vi "myRIO v1.0 Reset Encoder.vi"(8 "error in (no error)":errorcluster, 10 "Channel":T1, 11 "myRIO Ref In":T2) -> (0 "error out":errorcluster, 3 "myRIO Ref Out":T2)   [LabVIEW 2021]
uses:
  <vilib>/myRIO/Common/Instrument Driver Framework/Utilities/typedefs/myRIO v1.0 Reference.ctl
  <vilib>/myRIO/Common/Instrument Driver Framework/Utilities/typedefs/Generic FPGA Reference.ctl
  <vilib>/myRIO/Common/Instrument Driver Framework/myRIO v1.0/Encoder/typedefs/Encoder Channels Enum.ctl
  <vilib>/myRIO/Common/Instrument Driver Framework/myRIO v1.0/Encoder/typedefs/Encoder Channels FPGA Reference.ctl
  <vilib>/rvi/errors/niLvFpgaAdjustHostInterfaceError.vi
  <vilib>/rvi/interface/nirviReadWriteControl/nirviReadWriteControl.xnode
  <vilib>/rvi/interface/Simulation/niFpgaSimulationCallBeginRW.vi
  NiFpgaLv.dll
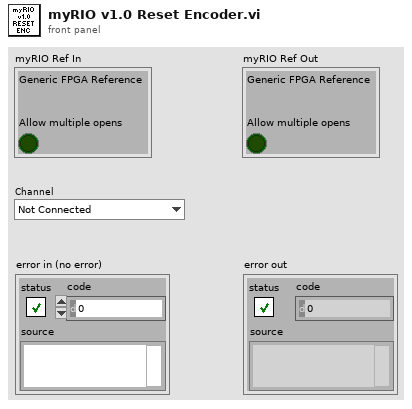
[diagram p1: front panel]
types:
  T1 = typedef "Encoder Channels Enum.ctl" = enum16{"Not Connected", "C/ENC0", "C/ENC1", "A/ENC", "A/ENC0", "A/ENC1", "A/ENC2", "A/ENC3", "A/ENC4", "A/ENC5", "A/ENC6", "A/ENC7", "A/ENC8", "A/ENC9", "B/ENC", "B/ENC0", "B/ENC1", "B/ENC2", "B/ENC3", "B/ENC4", "B/ENC5", "B/ENC6", "B/ENC7", "B/ENC8", "B/ENC9", "DIO/ENC0", "DIO/ENC1", "DIO/ENC2", "DIO/ENC3", "DIO/ENC4"}
  T2 = typedef "myRIO v1.0 Reference.ctl" = cluster{"Generic FPGA Reference":T3, "Allow multiple opens":bool}
  T3 = typedef "Generic FPGA Reference.ctl" = refnum<k20>
  T4 = typedef "Encoder Channels FPGA Reference.ctl" = refnum<k20>
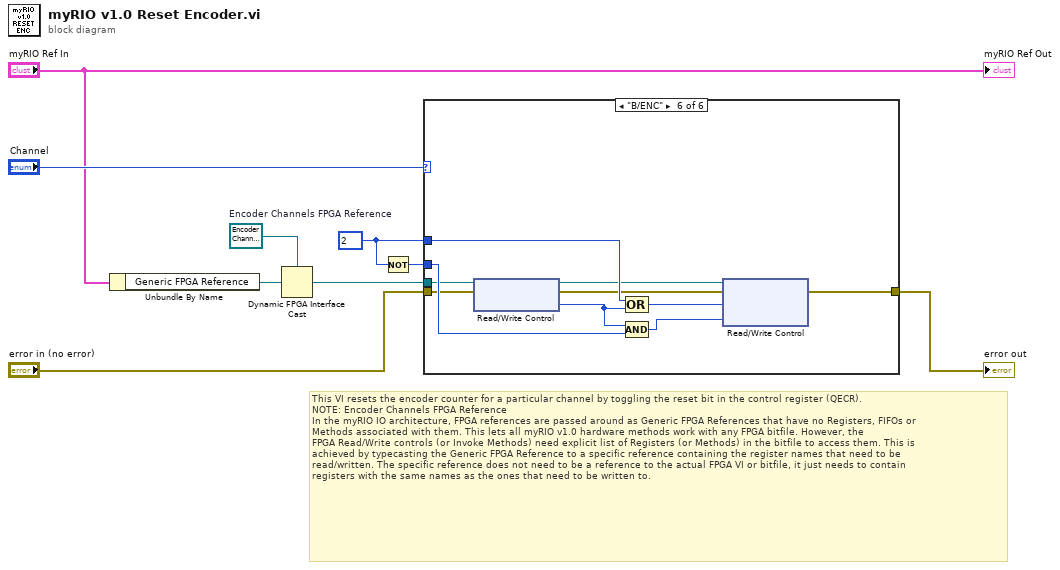
[diagram p0: block diagram]
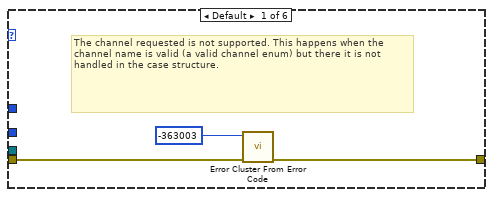
[diagram p2: hidden frame]
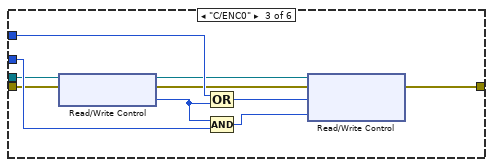
[diagram p4: hidden frame]
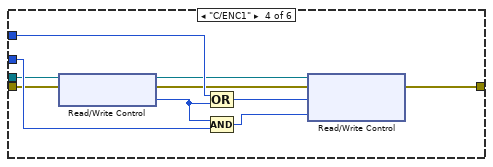
[diagram p5: hidden frame]
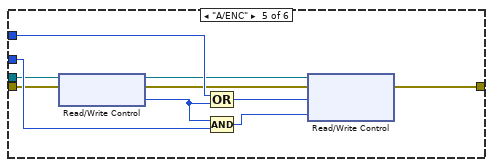
[diagram p6: hidden frame]
diagram:
  w4 = u8 2
  w9 = T4 refnum  # Encoder Channels FPGA Reference
  # "This VI resets the encoder counter for a particular channel by toggling the reset bit in the control register (QECR).\nNOTE: Encoder Channels FPGA Reference\nIn the myRIO IO architecture, FPGA references are passed around as Generic FPGA References that have no Registers, FIFOs or\nMethods associated with them. This lets all myRIO v1.0 hardware methods work with any FPGA bitfile. However, the \nFPGA Read/Write controls (or Invoke Methods) need explicit list of Registers (or Methods) in the bitfile to access them. This is \nachieved by typecasting the Generic FPGA Reference to a specific reference containing the register names that need to be \nread/written. The specific reference does not need to be a reference to the actual FPGA VI or bitfile, it just needs to contain \nregisters with the same names as the ones that need to be written to."
  n1 = Unbundle By Name("myRIO Ref In") -> ("Generic FPGA Reference"=w2:T3)
  n2 = Dynamic FPGA Interface Cast(Session In=w9, Type=w2) -> (Session Out=w8:T4)
  n3 = Not(x=w4) -> (.not. x?=w3:u8)
  n4 = case shown="\"B/ENC\"" "Channel" {
    tunnel: "error in (no error)" -> [w10 w13 w20 w30 w40 w50]
    tunnel: [w11 w13 w14 w24 w34 w44] -> w5
    tunnel: w8 -> [_ _ w21 w31 w41 w51]
    tunnel: w4 -> [_ _ w23 w33 w43 w53]
    tunnel: w3 -> [_ _ w22 w32 w42 w52]
    frame Default {
      # "The channel requested is not supported. This happens when the channel name is valid (a valid channel enum) but there it is not handled in the case structure."
      n5 = call <vilib>:"Error Cluster From Error Code.vi"("error in (no error)"=w10, "error code (0)"=-363003) -> ("error out"=w11:errorcluster)  [unwired: 7 in]
    }
    frame "Not Connected" {
    }
    frame "C/ENC0" {
      n6 = xnode "Read/Write Control"("FPGA VI Reference In"=w21, "error in"=w20) -> ("FPGA VI Reference Out"=w18:T4, "error out"=w17:errorcluster, "ENC.C_0.CNFG"=w19:u8)
      n7 = Compound Arithmetic op=OR(w23, w19) -> (w16:u8)
      n8 = Compound Arithmetic op=AND(w19, w22) -> (w15:u8)
      n9 = xnode "Read/Write Control"("FPGA VI Reference In"=w18, "error in"=w17, "ENC.C_0.CNFG"=w16, "ENC.C_0.CNFG"=w15) -> ("error out"=w14:errorcluster)  [unwired: 1 out]
    }
    frame "C/ENC1" {
      n10 = xnode "Read/Write Control"("FPGA VI Reference In"=w31, "error in"=w30) -> ("FPGA VI Reference Out"=w28:T4, "error out"=w27:errorcluster, "ENC.C_1.CNFG"=w29:u8)
      n11 = Compound Arithmetic op=OR(w33, w29) -> (w26:u8)
      n12 = Compound Arithmetic op=AND(w29, w32) -> (w25:u8)
      n13 = xnode "Read/Write Control"("FPGA VI Reference In"=w28, "error in"=w27, "ENC.C_1.CNFG"=w26, "ENC.C_1.CNFG"=w25) -> ("error out"=w24:errorcluster)  [unwired: 1 out]
    }
    frame "A/ENC" {
      n14 = xnode "Read/Write Control"("FPGA VI Reference In"=w41, "error in"=w40) -> ("FPGA VI Reference Out"=w38:T4, "error out"=w37:errorcluster, "ENC.A.CNFG"=w39:u8)
      n15 = Compound Arithmetic op=OR(w43, w39) -> (w36:u8)
      n16 = Compound Arithmetic op=AND(w39, w42) -> (w35:u8)
      n17 = xnode "Read/Write Control"("FPGA VI Reference In"=w38, "error in"=w37, "ENC.A.CNFG"=w36, "ENC.A.CNFG"=w35) -> ("error out"=w34:errorcluster)  [unwired: 1 out]
    }
    frame "B/ENC" {
      n18 = xnode "Read/Write Control"("FPGA VI Reference In"=w51, "error in"=w50) -> ("FPGA VI Reference Out"=w48:T4, "error out"=w47:errorcluster, "ENC.B.CNFG"=w49:u8)
      n19 = Compound Arithmetic op=OR(w53, w49) -> (w46:u8)
      n20 = Compound Arithmetic op=AND(w49, w52) -> (w45:u8)
      n21 = xnode "Read/Write Control"("FPGA VI Reference In"=w48, "error in"=w47, "ENC.B.CNFG"=w46, "ENC.B.CNFG"=w45) -> ("error out"=w44:errorcluster)  [unwired: 1 out]
    }
  }
  "error out" <- w5
  "myRIO Ref Out" <- "myRIO Ref In"
